vi "program_power_supply_gpib.vi"(1 "Power Supply Controls":T1={"+6V output Voltage"=6.0, "+6V output Current"=1.812, "+25V output Voltage"=25.0, "+25V output Current"=0.241} {"+25V output Current" format="%.3f"; "+25V output Voltage" format="%.3f"; "+6V output Current" format="%.3f"; "+6V output Voltage" format="%.3f"}, 2 "error in (no error)":errorcluster, 3 "Tracking(Off:F)":bool, 4 "Trigger(GPIB Bus:1)":u16(ring)=1 items=["Internal", "GPIB Bus"], 5 "GPIB Address (5)":i16=5) -> (0 "error out":errorcluster)   [LabVIEW 2013]
doc: "This VI allows the setting of the +6V and +25V outputs. It is not sufficient to set only the voltage or the current that is desired; set both at the approximate desired values for the power supply to correctly register them. Typically, the current will be set, and the voltage is whatever it takes to achieve that current."
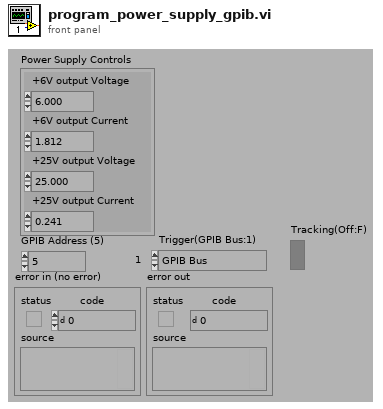
[diagram p1: front panel]
types:
  T1 = cluster{"+6V output Voltage":dbl, "+6V output Current":dbl, "+25V output Voltage":dbl, "+25V output Current":dbl}
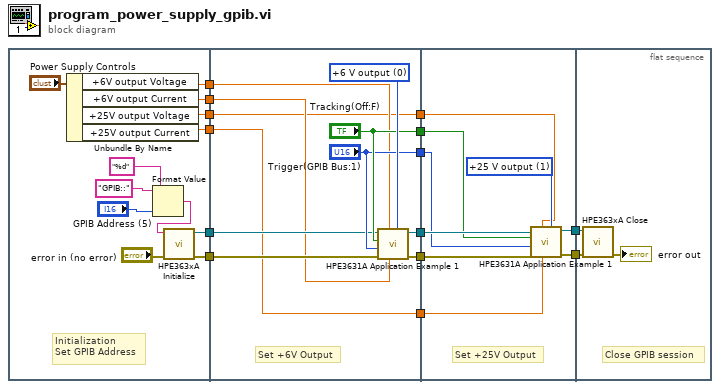
[diagram p0: block diagram]
diagram:
  n1 = flat-sequence {
    tunnel: [w22] -> w8
    tunnel: [w23] -> w7
    tunnel: [w18] -> w6
    tunnel: [w17] -> w5
    tunnel: [w16] -> w3
    tunnel: [w15] -> w1
    tunnel: ["Tracking(Off:F)"] -> w14
    tunnel: ["Trigger(GPIB Bus:1)"] -> w13
    tunnel: [w34] -> w12
    tunnel: [w33] -> w10
    tunnel: w8 -> [w31]
    tunnel: w7 -> [w32]
    tunnel: w6 -> [w30]
    tunnel: w5 -> [w29]
    tunnel: [w28] -> w4
    tunnel: w3 -> [w28]
    tunnel: [w27] -> w2
    tunnel: w1 -> [w27]
    tunnel: w14 -> [w40]
    tunnel: w13 -> [w41]
    tunnel: w12 -> [w46]
    tunnel: [w45] -> w11
    tunnel: w10 -> [w43]
    tunnel: [w42] -> w9
    tunnel: w4 -> [w39]
    tunnel: w2 -> [w38]
    tunnel: w11 -> [w48]
    tunnel: w9 -> [w47]
    frame #0 {
      # "Initialization\nSet GPIB Address"
      n2 = Unbundle By Name("Power Supply Controls") -> ("+6V output Voltage"=w18:dbl, "+6V output Current"=w17:dbl, "+25V output Voltage"=w16:dbl, "+25V output Current"=w15:dbl)
      n3 = Format Value(string ("")="GPIB::", format string="%d", value (0)="GPIB Address (5)") -> (output string=w20:string)
      n4 = call "HPE363xA Initialize.vi"("error in (no error)"="error in (no error)", "Instr. Descriptor (GPIB::5)"=w20) -> ("error in (no error)"=w22:errorcluster, "VISA session"=w23:refnum<visa-resource-name>)  [unwired: 8 in]
    }
    frame #1 {
      w37 = u16 0 items=["+6 V output", "+25 V output", "-25 V output"] ("Output Terminals(+6 V:0)")
      # "Set +6V Output"
      n5 = call "HPE3631A Application Example 1.vi"("Output Terminals(+6 V:0)"=w37, "Current(0)"=w29, "Voltage(0)"=w30, "error in (no error)"=w31, "Trigger(GPIB Bus:1)"="Trigger(GPIB Bus:1)", "Tracking(Off:F)"="Tracking(Off:F)", "VISA session"=w32) -> ("error out"=w34:errorcluster, "dup VISA session"=w33:refnum<visa-resource-name>)  [unwired: 2 in]
    }
    frame #2 {
      w44 = u16 1 items=["+6 V output", "+25 V output", "-25 V output"] ("Output Terminals(+6 V:0)")
      # "Set +25V Output"
      n6 = call "HPE3631A Application Example 1.vi"("Output Terminals(+6 V:0)"=w44, "Current(0)"=w38, "Voltage(0)"=w39, "error in (no error)"=w46, "Trigger(GPIB Bus:1)"=w41, "Tracking(Off:F)"=w40, "VISA session"=w43) -> ("error out"=w45:errorcluster, "dup VISA session"=w42:refnum<visa-resource-name>)  [unwired: 2 in]
    }
    frame #3 {
      # "Close GPIB session"
      n7 = call "HPE363xA Close.vi"("error in (no error)"=w48, "VISA session"=w47) -> ("error out"=→"error out":errorcluster)  [unwired: 9 in]
    }
  }
